vi "Average.vi"(8 "error in (no error)":errorcluster, 10 "Configure":T1={"X Low"=0.05, "X High"=0.5, "X Step"=0.01, "Fake Point"=0.05} {"Fake Point" format="%#_6p"; "X Step" format="%#_6p"; "X High" format="%#_6p"; "X Low" format="%#_6p"}, 11 "XY-data":cluster{"X-array":dbl[], "Y-array":dbl[]}[](array[cluster]) {"Y-array" format="%.2p"; "X-array" format="%.2p"}) -> (0 "error out":errorcluster, 2 "Averaged XY-data out":cluster{"X-array":dbl[], "Y-array":dbl[]} {"Y-array" format="%.2p"; "X-array" format="%.2p"}, 3 "XY-data out":cluster{"X-array":dbl[], "Y-array":dbl[]}[](array[cluster]) {"Y-array" format="%.2p"; "X-array" format="%.2p"})   [LabVIEW 2019, in "xy_utilities.lvlib"]
doc: "Calculates the <b>Mean</b> of the y arrays in <b>XY-data</b> at x values defined by the <b>Configure</b> Cluster.\n\n<b>XY-data</b> is not assumed to have commensurate x values or sampling; therefore interpolation is performed before averaging.\n\nThe <b>Configure</b> cluster is used to define:\n<b>X Low</b>: Starting x value for interpolation. May lie outside of the input x array range.\n<b>X High</b>: Ending x value for interpolation. May lie outside of the input x array range.\n<b>X Step</b>: Interpolation value.\n<b>Fake Point</b>: Value added to the y array for x values outside of the x array input range.\n\nNote that this VI returns two types of data:\n<b>XY-data out</b> is the original input data array <b>XY-data</b>.\n<b>Averaged XY-data out</b> is a single containing the averaged XY-data.\n\nNote also that this is NOT a polymorphic VI. It will only work for an input that is an array of XY-data."
uses:
  xy_utilities.lvlib
  <vilib>/Analysis/NI_AALBase.lvlib
  <vilib>/Analysis/baseanly.llb/Mean (DBL).vi
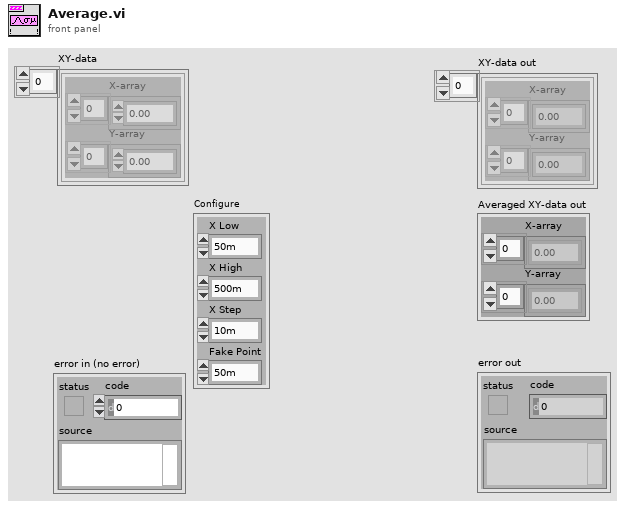
[diagram p1: front panel]
types:
  T1 = cluster{"X Low":dbl, "X High":dbl, "X Step":dbl, "Fake Point":dbl}
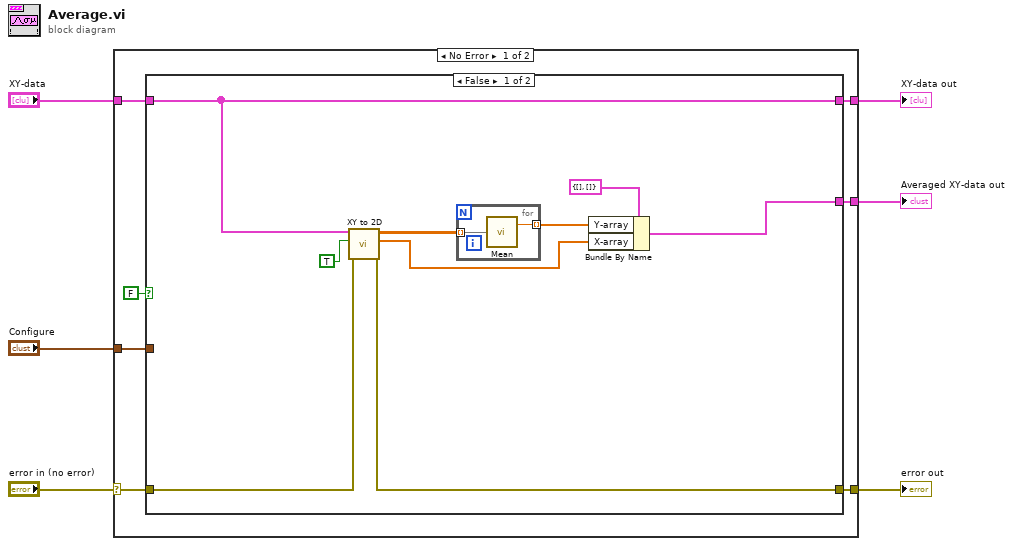
[diagram p0: block diagram]
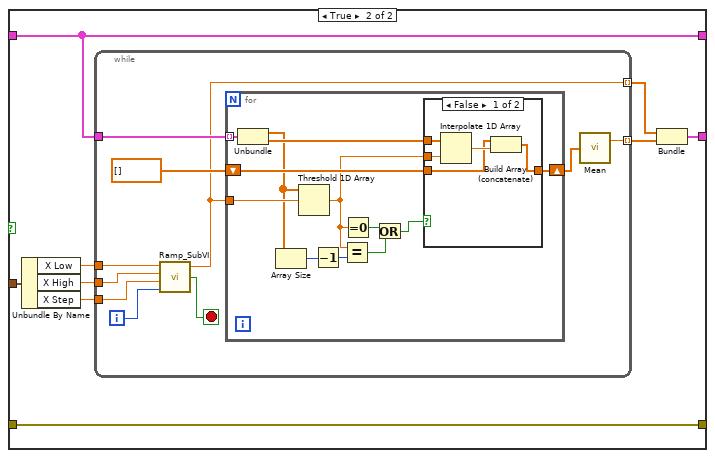
[diagram p2: hidden frame]
diagram:
  n1 = case shown="No Error" "error in (no error)" {
    selector: "error in (no error)" -> [w9 w62]
    tunnel: [w7 w63] -> w6
    tunnel: "XY-data" -> [w11 w63]
    tunnel: [w8 w62] -> w5
    tunnel: "Configure" -> [w13 _]
    tunnel: [w12 _] -> w3
    frame No Error {
      n2 = case shown="False" FALSE {
        tunnel: w13 -> [_ w32]
        tunnel: [w17 w27] -> w12
        tunnel: w11 -> [w16 w26]
        tunnel: w9 -> [w19 w25]
        tunnel: [w18 w25] -> w8
        tunnel: [w16 w26] -> w7
        frame False {
          n3 = call "XY to 2D.vi"("error in (no error)"=w19, "Interpolate [T]"=TRUE, "XY-data"=w16) -> ("error out"=w18:errorcluster, "X Array"=w22:dbl[], "2D Y Array"=w14:dbl[][])  [unwired: 5 in, 1 out]
          n4 = for {
            tunnel: w14 -> [w24] mode=indexing
            tunnel: [w23] -> w21 mode=indexing
            n5 = call-poly <vilib>:"Mean.vi"("X"=w24) -> ("mean"=w23:dbl)  [unwired: 1 out]
          }
          n6 = Bundle By Name(cluster=cluster{"X-array":dbl[], "Y-array":dbl[]} {"X-array"=[], "Y-array"=[]}, "Y-array"=w21, "X-array"=w22) -> (w17:cluster{"X-array":dbl[], "Y-array":dbl[]})
        }
        frame True {
          n7 = Unbundle By Name(w32) -> ("X Low"=w31:dbl, "X High"=w30:dbl, "X Step"=w28:dbl)
          n8 = while {
            tunnel: [w42] -> w33 mode=indexing
            tunnel: [w39] -> w29 mode=indexing
            tunnel: w26 -> [w40]
            tunnel: w31 -> [w38]
            tunnel: w30 -> [w37]
            tunnel: w28 -> [w36]
            i -> [w35]
            stop <- w34 stop-if-true
            n9 = call "Ramp_SubVI.vi"("index"=w35, "step"=w36, "end"=w37, "start"=w38) -> ("Stop?"=w34:bool, "Numeric"=w39:dbl)  [unwired: 1 in]
            n10 = for {
              tunnel: w40 -> [w55] mode=indexing
              shift-right: [w54] -> w41
              shift-left: dbl[] [] -> [w53]
              tunnel: w39 -> [w52]
              n11 = Unbundle(w55) -> ("X-array"=w45:dbl[], "Y-array"=w46:dbl[])
              n12 = Array Size(array=w45) -> (size(s)=w48:i32)
              n13 = Threshold 1D Array(2:w52, 3:w45) -> (0:w50:dbl)  [unwired: 1 in]
              n14 = Decrement(x=w48) -> (x-1=w47:i32)
              n15 = Equal?(x=w50, y=w47) -> (x = y?=w49:bool)
              n16 = Equal To 0?(x=w50) -> (x = 0?=w51:bool)
              n17 = Or(x=w51, y=w49) -> (x .or. y?=w44:bool)
              n18 = case shown="False" w44 {
                tunnel: [w58 w61] -> w54
                tunnel: w50 -> [w60 _]
                tunnel: w46 -> [w59 _]
                tunnel: w53 -> [w56 w61]
                frame False {
                  n19 = Interpolate 1D Array(1:w60, 2:w59) -> (0:w57:dbl)
                  n20 = Build Array (concatenate)(w56, w57) -> (w58:dbl[])
                }
                frame True {
                }
              }
            }
            n21 = call-poly <vilib>:"Mean.vi"("X"=w41) -> ("mean"=w42:dbl)  [unwired: 1 out]
          }
          n22 = Bundle(w29, w33) -> (w27:cluster{dbl[], dbl[]})  [unwired: 1 in]
        }
      }
    }
    frame Error {
    }
  }
  "XY-data out" <- w6
  "error out" <- w5
  "Averaged XY-data out" <- w3
